vi "Run Simple Data Acquisition.vi"(4 "Thresholding Cluster":T1={"F_DEx"=0, "F_AA"=0, " No of Bins"=100}, 5 "output cluster 2":T2, 6 "Files To Acquire Refnum":refnum<vi>, 7 "Path Refnum":refnum<vi>, 8 "error in":errorcluster, 9 "Data File I/O Information":T3={"Name of Configuration"="", "Path"=path "C:/Users/Achilles/Data/12-20-00", "File Name"="Whole Gel Image", "Files To Acquire"=1, "Current File Number"=21, "Time Limit"=1.0, "Save Data"=FALSE, "Additional Comments"=""}, 10 "Time Limit":dbl=1.0, 11 "File Type":string) -> (0 "error in 2":errorcluster, 1 "Data File I/O Information":T3={"Name of Configuration"="", "Path"=path "C:/Users/Achilles/Data/12-20-00", "File Name"="Whole Gel Image", "Files To Acquire"=1, "Current File Number"=21, "Time Limit"=1.0, "Save Data"=FALSE, "Additional Comments"=""})   [LabVIEW 2009]
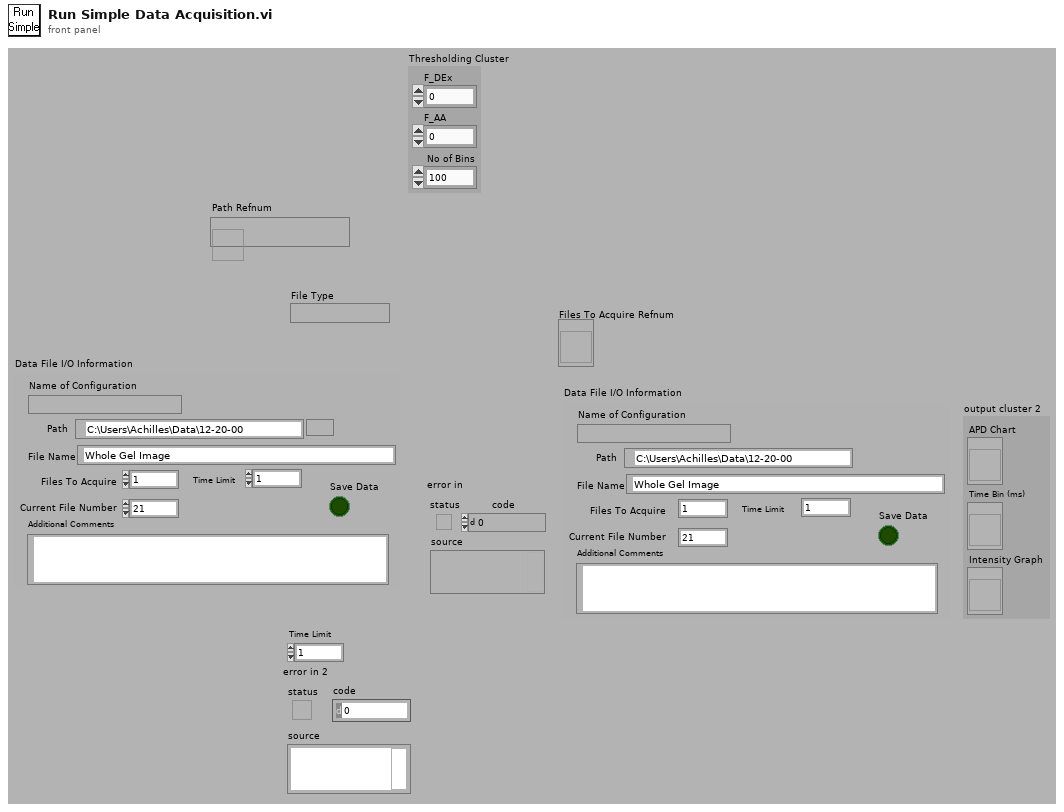
[diagram p1: front panel]
types:
  T1 = cluster{"F_DEx":i32, "F_AA":i32, " No of Bins":i32}
  T2 = cluster{"APD Chart":refnum<vi>, "Time Bin (ms)":refnum<vi>, "Intensity Graph":refnum<vi>}
  T3 = cluster{"Name of Configuration":string, "Path":path, "File Name":string, "Files To Acquire":i32, "Current File Number":i32, "Time Limit":dbl, "Save Data":bool, "Additional Comments":string}
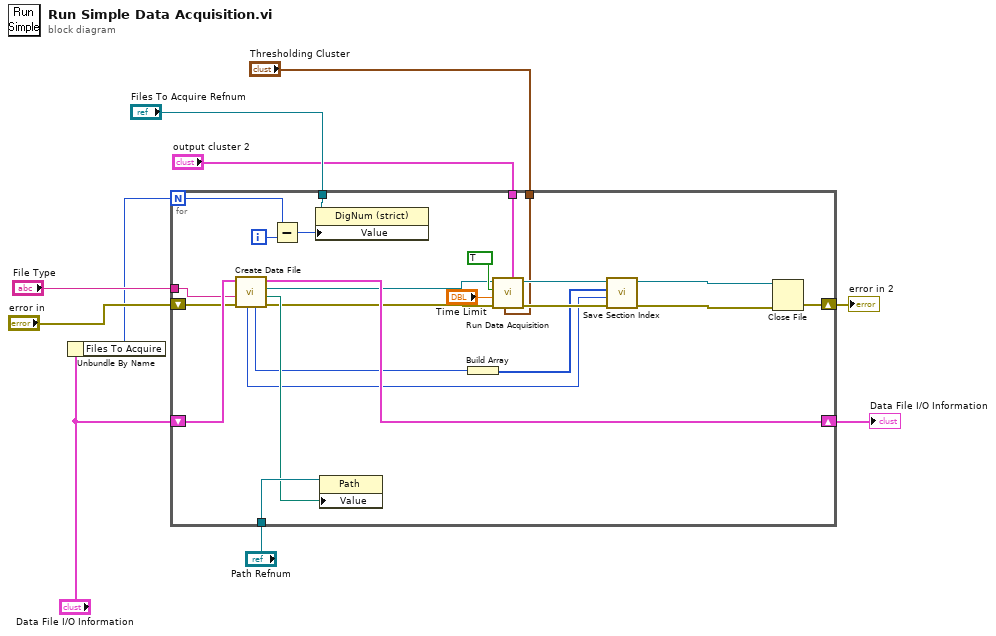
[diagram p0: block diagram]
diagram:
  n1 = Unbundle By Name("Data File I/O Information") -> ("Files To Acquire"=w6:i32)
  n2 = for {
    N: w6 -> [w34]
    shift-right: [w24] -> w3
    shift-left: "error in" -> [w31]
    shift-right: [w30] -> w9
    shift-left: "Data File I/O Information" -> [w32]
    tunnel: "File Type" -> [w16]
    tunnel: "Path Refnum" -> [w28]
    tunnel: "Files To Acquire Refnum" -> [w25]
    tunnel: "output cluster 2" -> [w12]
    tunnel: "Thresholding Cluster" -> [w11]
    i -> [w33]
    n3 = call "Create Data File.vi"("error in (no error)"=w31, "File Type"=w16, "Data File I/O Information"=w32) -> ("error out"=w15:errorcluster, "new file path"=w27:path, "refnum"=w14:refnum<file>, "Data File I/O Information"=w30:T3, "First section offset"=w18:i32, "Offset for index pointer"=w17:i32)  [unwired: 3 in]
    n4 = Subtract(x=w34, y=w33) -> (x-y=w26:i32)
    n5 = property class="DigNum (strict)"(reference=w25, "Value"=w26) -> ()  [unwired: 1 in, 2 out]
    n6 = property class="Path"(reference=w28, "Value"=w27) -> ()  [unwired: 1 in, 2 out]
    n7 = Build Array(w18) -> (w19:i32[])
    n8 = call "Run Data Acquisition.vi"("output cluster 2"=w12, "Thresholding Cluster 2"=w11, "error in (no error)"=w15, "Time Limit"="Time Limit", "Save Data"=TRUE, "refnum in"=w14) -> ("error out"=w22:errorcluster, "refnum out"=w23:refnum<file>)  [unwired: 4 in]
    n9 = call "Save Section Index.vi"("error in (no error)"=w22, "Offset for index pointer"=w17, "File Section Offset"=w19, "refnum"=w23) -> ("error out"=w21:errorcluster, "dup refnum"=w20:refnum<file>)  [unwired: 6 in]
    n10 = Close File(refnum=w20, error in=w21) -> (error out=w24:errorcluster)  [unwired: 1 out]
  }
  "Data File I/O Information" <- w9
  "error in 2" <- w3
